vi "Initialize.vi"(0 "VISA resource name":refnum<visa-resource-name>, 1 "Error Queue Option":enum16{"Clear Error Queue", "Error Query"}(ring), 5 "RS-232 Settings":T1={"Read Term Char"=enum."CR", "Baud Rate"=enum."9600", "Flow Control\n(XON / XOFF)"=enum."Off"}, 11 "error in (no error)":errorcluster, 12 "ID Query? (T)":bool=TRUE, 13 "Reset? (T)":bool=TRUE) -> (4 "VISA resource name out":refnum<visa-resource-name>, 15 "error out":errorcluster)   [LabVIEW 2014, in "KE6514Driver.lvlib"]
doc: "Establishes communication with the instrument and optionally performs an instrument identification query and/or an instrument reset. Therefore, call this VI before calling other instrument driver VIs for this instrument. Generally, you need to call the Initialize VI only once at the beginning of an application."
uses:
  KE6514Driver.lvlib
panel:
  # "(c) 2010 Keithley Instruments.  ALL RIGHTS RESERVED."
  # "Serial settings must match those on the physical instrument.  Hardware flow control is not supported, but software flow control is (XON/XOFF)."
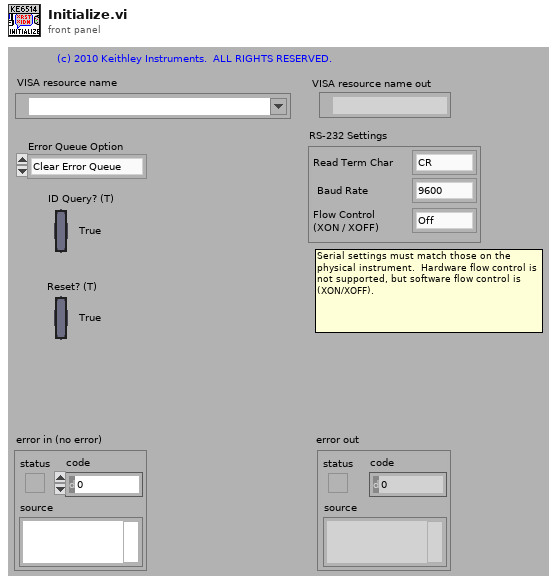
[diagram p1: front panel]
types:
  T1 = cluster{"Read Term Char":enum16{"CR", "LF", "CR + LF", "LF + CR"}, "Baud Rate":enum16{"300", "600", "1200", "2400", "4800", "9600", "19200", "38400", "57600"}, "Flow Control\n(XON / XOFF)":enum16{"Off", "On"}}
  T2 = enum16{"300", "600", "1200", "2400", "4800", "9600", "19200", "38400", "57600"}
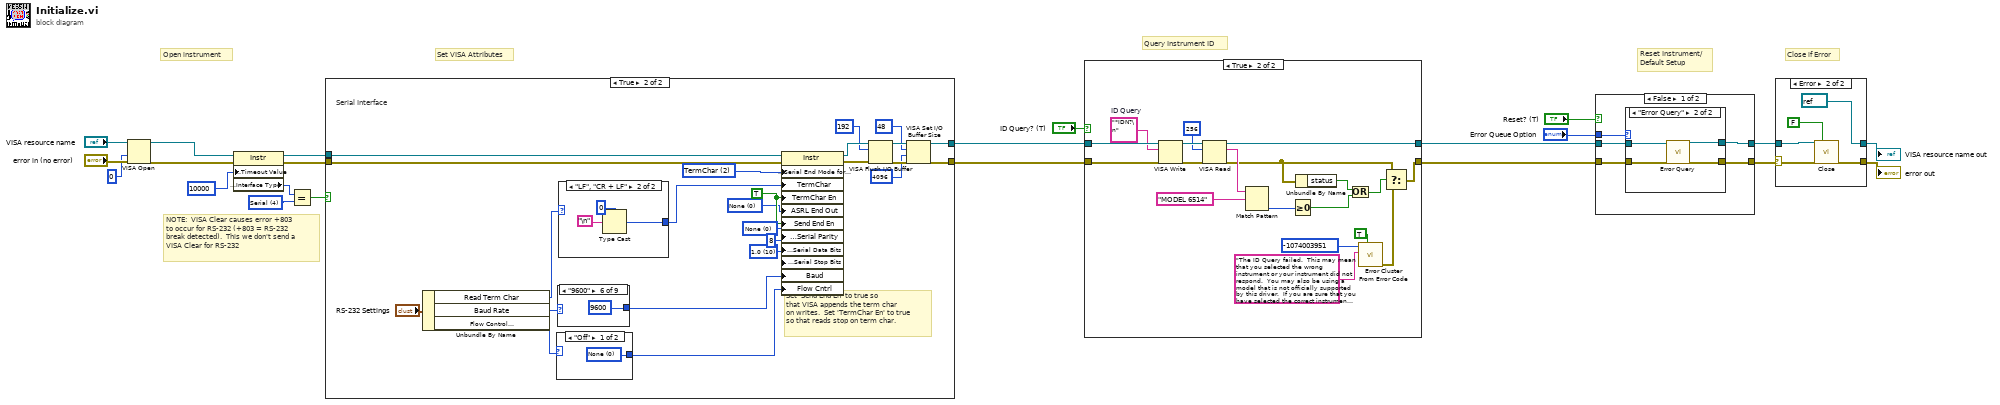
[diagram p0: block diagram]
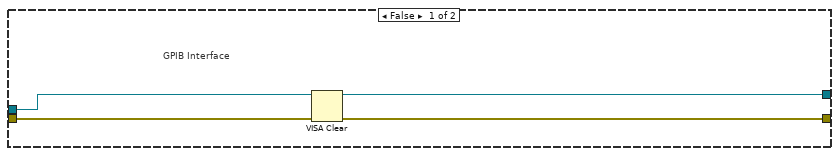
[diagram p2: hidden frame]
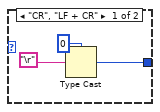
[diagram p3: hidden frame]
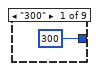
[diagram p4: hidden frame]
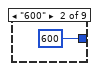
[diagram p5: hidden frame]
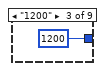
[diagram p6: hidden frame]
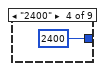
[diagram p7: hidden frame]
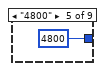
[diagram p8: hidden frame]
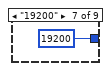
[diagram p9: hidden frame]
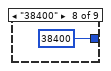
[diagram p10: hidden frame]
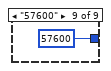
[diagram p11: hidden frame]
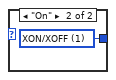
[diagram p12: hidden frame]
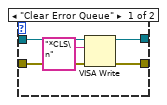
[diagram p14: hidden frame]
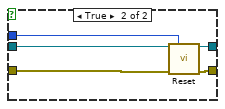
[diagram p15: hidden frame]
diagram:
  w10 = u16 4 items=["GPIB"=1, "VXI"=2, "GPIB-VXI"=3, "Serial"=4, "PXI"=5, "TCPIP"=6, "USB"=7] ("Interface Information:Interface Type")
  # "NOTE:  VISA Clear causes error +803\nto occur for RS-232 (+803 = RS-232\nbreak detected).  This we don't send a\nVISA Clear for RS-232"
  # "Set VISA Attributes"
  # "Close if Error"
  # "Query Instrument ID"
  # "Reset Instrument/\nDefault Setup"
  # "Open instrument"
  n1 = VISA Open(access mode=u32 0, error in (no error)="error in (no error)", VISA resource name="VISA resource name") -> (VISA resource name=w4:refnum<visa-resource-name>, error out=w3:errorcluster)  [unwired: 2 in]
  n2 = property class="Instr"(reference=w4, error in=w3, "General Settings:Timeout Value"=u32 10000) -> (reference out=w13:refnum<visa-resource-name>, error out=w12:errorcluster, "Interface Information:Interface Type"=w1:u16)
  n3 = Equal?(x=w1, y=w10) -> (x = y?=w11:bool)
  n4 = case shown="True" w11 {
    tunnel: [w23 w47] -> w15
    tunnel: [w24 w44] -> w14
    tunnel: w13 -> [w25 w49]
    tunnel: w12 -> [w26 w50]
    frame False {
      # "GPIB Interface"
      n5 = VISA Clear(VISA resource name=w25, error in (no error)=w26) -> (VISA resource name out=w23:refnum<visa-resource-name>, error out=w24:errorcluster)
    }
    frame True {
      w28 = u16 0 items=["None", "Last Bit", "TermChar", "Break"] ("Serial Settings:End Mode for Writes")
      w31 = TRUE ("Message Based Settings:Termination Character Enable")
      w32 = u16 2 items=["None", "Last Bit", "TermChar"] ("Serial Settings:End Mode for Reads")
      w37 = u16 10 items=["1.0"=10, "1.5"=15, "2.0"=20] ("Serial Settings:Stop Bits")
      w39 = u16 0 items=["None", "Odd", "Even", "Mark", "Space"] ("Serial Settings:Parity")
      # "Set 'Send End En' to true so\nthat VISA appends the term char\non writes.  Set 'TermChar En' to true\nso that reads stop on term char."
      # "Serial Interface"
      n6 = Unbundle By Name("RS-232 Settings") -> ("Read Term Char"=w34:enum16{"CR", "LF", "CR + LF", "LF + CR"}, "Baud Rate"=w35:T2, "Flow Control\n(XON / XOFF)"=w36:enum16{"Off", "On"})
      n7 = case shown="\"Off\"" w36 {
        tunnel: [w66 w67] -> w29
        frame "Off" {
          w66 = u16 0 items=["None", "XON/XOFF", "RTS/CTS", "XON/XOFF & RTS/CTS", "DTR/DSR", "XON/XOFF & DTR/DSR"] ("Serial Settings:Flow Control")
        }
        frame "On" {
          w67 = u16 1 items=["None", "XON/XOFF", "RTS/CTS", "XON/XOFF & RTS/CTS", "DTR/DSR", "XON/XOFF & DTR/DSR"] ("Serial Settings:Flow Control")
        }
      }
      n8 = case shown="\"9600\"" w35 {
        tunnel: [u32 300 ("Serial Settings:Baud Rate") u32 600 ("Serial Settings:Baud Rate") u32 1200 ("Serial Settings:Baud Rate") u32 2400 ("Serial Settings:Baud Rate") u32 4800 ("Serial Settings:Baud Rate") u32 9600 ("Serial Settings:Baud Rate") u32 19200 ("Serial Settings:Baud Rate") u32 38400 ("Serial Settings:Baud Rate") u32 57600 ("Serial Settings:Baud Rate")] -> w30
        frame "300" {
        }
        frame "600" {
        }
        frame "1200" {
        }
        frame "2400" {
        }
        frame "4800" {
        }
        frame "9600" {
        }
        frame "19200" {
        }
        frame "38400" {
        }
        frame "57600" {
        }
      }
      n9 = case shown="\"LF\", \"CR + LF\"" w34 {
        tunnel: [w51 w55] -> w33
        frame "CR", "LF + CR" {
          n10 = Type Cast(type=u8 0, x="\r") -> (*(type *) &x=w51:u8)
        }
        frame "LF", "CR + LF" {
          n11 = Type Cast(type=u8 0, x="\n") -> (*(type *) &x=w55:u8)
        }
      }
      n12 = property class="Instr"(reference=w49, error in=w50, "Serial Settings:Serial End Mode for Reads"=w32, "TermChar"=w33, "TermChar En"=w31, "ASRL End Out"=w28, "Send End En"=w31, "Serial Settings:Serial Parity"=w39, "Serial Settings:Serial Data Bits"=u16 8 ("Serial Settings:Data Bits"), "Serial Settings:Serial Stop Bits"=w37, "Baud"=w30, "Flow Cntrl"=w29) -> (reference out=w43:refnum<visa-resource-name>, error out=w46:errorcluster)
      n13 = VISA Flush I/O Buffer(VISA resource name=w43, mask (16)=u16 192, error in (no error)=w46) -> (VISA resource name out=w48:refnum<visa-resource-name>, error out=w45:errorcluster)
      n14 = VISA Set I/O Buffer Size(VISA resource name=w48, mask (16)=u16 48, size (4096)=u32 4096 ("size (0)"), error in (no error)=w45) -> (VISA resource name out=w47:refnum<visa-resource-name>, error out=w44:errorcluster)
    }
  }
  n15 = case shown="True" "ID Query? (T)" {
    tunnel: [w68 w88] -> w21
    tunnel: [w69 w85] -> w22
    tunnel: w15 -> [w69 w86]
    tunnel: w14 -> [w68 w87]
    frame False {
    }
    frame True {
      w80 = "*IDN?\n"  # ID Query
      n16 = VISA Write(VISA resource name=w86, write buffer=w80, error in (no error)=w87) -> (VISA resource name out=w83:refnum<visa-resource-name>, error out=w82:errorcluster)  [unwired: 1 out]
      n17 = VISA Read(VISA resource name=w83, byte count=u32 256, error in (no error)=w82) -> (VISA resource name out=w85:refnum<visa-resource-name>, read buffer=w84:string, error out=w74:errorcluster)  [unwired: 1 out]
      n18 = Match Pattern(string=w84, regular expression="MODEL 6514") -> (offset past match=w75:i32)  [unwired: 1 in, 3 out]
      n19 = Greater Or Equal To 0?(x=w75) -> (x >= 0?=w72:bool)
      n20 = Unbundle By Name(w74) -> ("status"=w73:bool)
      n21 = Or(x=w73, y=w72) -> (x .or. y?=w71:bool)
      n22 = call <vilib>:"Error Cluster From Error Code.vi"("show call chain? (False)"=TRUE, "error message (\"\")"="The ID Query failed.  This may mean that you selected the wrong instrument or your instrument did not respond.  You may also be using a model that is not officially supported by this driver.  If you are sure that you have selected the correct instrument and it is responding, try disabling the ID Query." ("Source (VI Name)"), "error code (0)"=-1074003951 ("Code")) -> ("error out"=w79:errorcluster)  [unwired: 6 in]
      n23 = Select(t=w74, s=w71, f=w79) -> (s? t:f=w88:errorcluster)
    }
  }
  n24 = case shown="False" "Reset? (T)" {
    tunnel: w21 -> [w90 w106]
    tunnel: [w92 w105] -> w5
    tunnel: w22 -> [w91 w107]
    tunnel: [w93 w104] -> w6
    tunnel: "Error Queue Option" -> [w89 w103]
    frame False {
      n25 = case shown="\"Error Query\"" w89 {
        tunnel: [w95 w102] -> w93
        tunnel: [w96 w101] -> w92
        tunnel: w91 -> [w98 w100]
        tunnel: w90 -> [w97 w99]
        frame "Clear Error Queue" {
          n26 = VISA Write(VISA resource name=w98, write buffer="*CLS\n", error in (no error)=w97) -> (VISA resource name out=w95:refnum<visa-resource-name>, error out=w96:errorcluster)  [unwired: 1 out]
        }
        frame "Error Query" {
          n27 = call "Error Query.vi"("VISA Resource In"=w100, "error in (no error)"=w99) -> ("VISA Resource Out (dupl)"=w102:refnum<visa-resource-name>, "error out"=w101:errorcluster)  [unwired: 10 in, 2 out]
        }
      }
    }
    frame True {
      n28 = call "Reset.vi"("VISA resource name"=w107, "Error Queue Option"=w103, "error in (no error)"=w106) -> ("VISA resource name out"=w104:refnum<visa-resource-name>, "error out"=w105:errorcluster)  [unwired: 11 in]
    }
  }
  n29 = case shown="Error" w5 {
    selector: w5 -> [w108 w112]
    tunnel: w6 -> [w109 w113]
    tunnel: [w109 refnum<visa-resource-name> refnum ("VISA resource name out")] -> w8
    tunnel: [w108 w114] -> w7
    frame No Error {
    }
    frame Error {
      n30 = call "Close.vi"("VISA resource name"=w113, "Query For SCPI Errors? (T)"=FALSE, "error in (no error)"=w112) -> ("error out"=w114:errorcluster)  [unwired: 12 in]
    }
  }
  "VISA resource name out" <- w8
  "error out" <- w7
